vi "rpc_tsmaster_call_library_api.vi"(4 "AArgs":string, 6 "AArgCount":i32, 7 "AArgCapacity":i32, 8 "error in (no error)":errorcluster caption="错误输入（无错误）", 9 "AHandle":u32, 10 "AAPIName":string, 11 "路径输入":path) -> (0 "error out":errorcluster caption="错误输出", 2 "function return":i32, 3 "路径输出":path)   [LabVIEW 2014]
doc: "TSAPI(s32)rpc_tsmaster_call_library_api(const size_t AHandle,const char* AAPIName,const s32 AArgCount,const s32 AArgCapacity,const ppchar AArgs);"
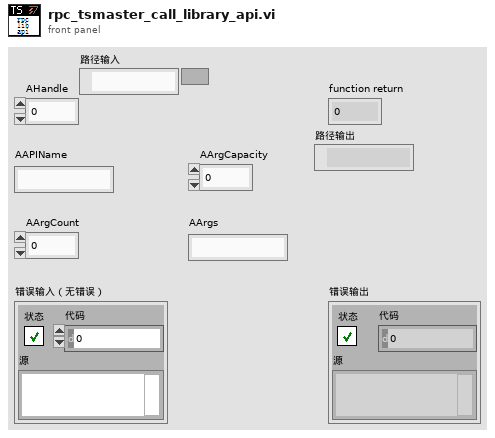
[diagram p1: front panel]
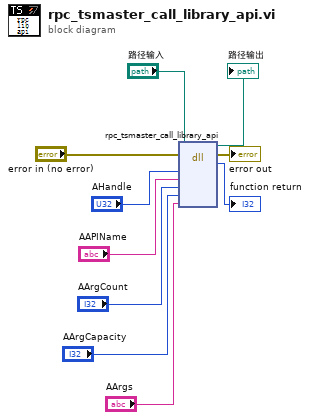
[diagram p0: block diagram]
diagram:
  n1 = dll-call lib="D:/Work/LabVIEW Code/TSMaster Labview SDK/LabVIEW/LabVIEW-TSMasterAPI_CLN/TSMasterAPI_LabVIEW-2024-10-08 14-20-13/Not_organized_vi/TSMaster.*" fn="rpc_tsmaster_call_library_api"(path in="路径输入", error in="error in (no error)", "AHandle"="AHandle", "AAPIName"="AAPIName", "AArgCount"="AArgCount", "AArgCapacity"="AArgCapacity", "AArgs"="AArgs") -> (path out=→"路径输出":path, error out=→"error out":errorcluster, "返回类型"=→"function return":i32)  [unwired: 6 in]
